vi "Constants.vi"() -> ()   [LabVIEW 2020, in "MIL-STD 1553 Import.lvlib"]
uses:
  MIL-STD 1553 Import.lvlib
panel:
  in  "terminals":string="terminals"
  in  "create trigger channel":string="createTriggerChannel"
  in  "acyclic frame":string="acyclicFrame"
  in  "direction":string="direction"
  in  "channel":string="channel"
  in  "hardware channel":string="hardwareChannel"
  in  "message":string="message"
  in  "create timestamp channel":string="createTimestampChannel"
  in  "subaddress":string="subAddress"
  in  "terminal address":string="terminalAddress"
  in  "number of words":string="numberOfWords"
  in  "mode Code":string="modeCode"
  in  "address":string="address"
  in  "message type":string="messageType"
  in  "parameter":string="parameter"
  in  "unit":string="unit"
  in  "offset":string="offset"
  in  "scale":string="scale"
  in  "signed":string="signed"
  in  "encoding":string="encoding"
  in  "size":string="numberOfBits"
  in  "start index":string="startBit"
  in  "default value":string="defaultValue"
  in  "name":string="name"
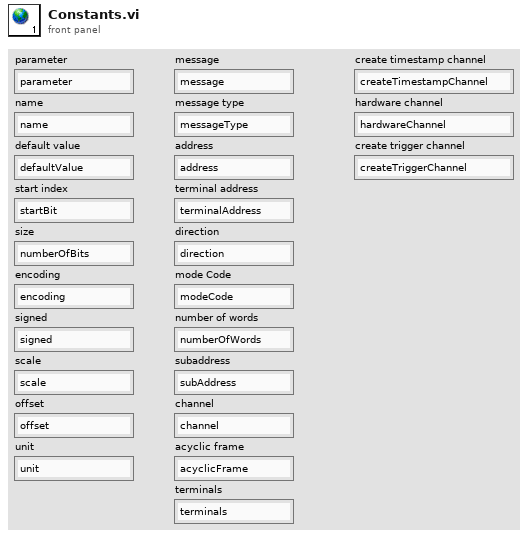
[diagram p1: front panel]
diagram:
